vi "TEB.vi"() -> ()   [LabVIEW 2019]
doc: "This is the Target Event Builder (TEB). It basically sits around and waits for event fragments to come in. Each fragment also has an event number attached to it. The TEB stores all fragments indexded by their associated eventnum.\nThe TEB sends fragments to any module appearing in the TEB config file's list. Each destination module can specify what fragments it wants and when those fragments should be sent. The \"when\" decision is made by the TEB based on the age of a given event, the age being determined by how many later events have come in.\nFor example, a module that saves data to disk might specify that it wants its data to be sent after it's 2 events old. So once data for event #1 comes in, it sits in the TEB buffer. Next, data for event #2 comes in, but the TEB keeps the event #1 data in its buffer. Only after event #3 is started (thereby making the event #1 data 2 events old) would the TEB ship event #1 to the module. This aging scheme was added when it was realized that some data for a given event (such as on-line analysis results) may be dependent on sucessive events, and therefore the data cannot be saved until those later events have also started to come in."
uses:
  TEB Global.vi
panel:
  out "Module Response":refnum<k4>
  out "Begin Post Processing":refnum<k4>
  out "Previous Event":T1
  out "Current Event":T1
  in  "stop":bool
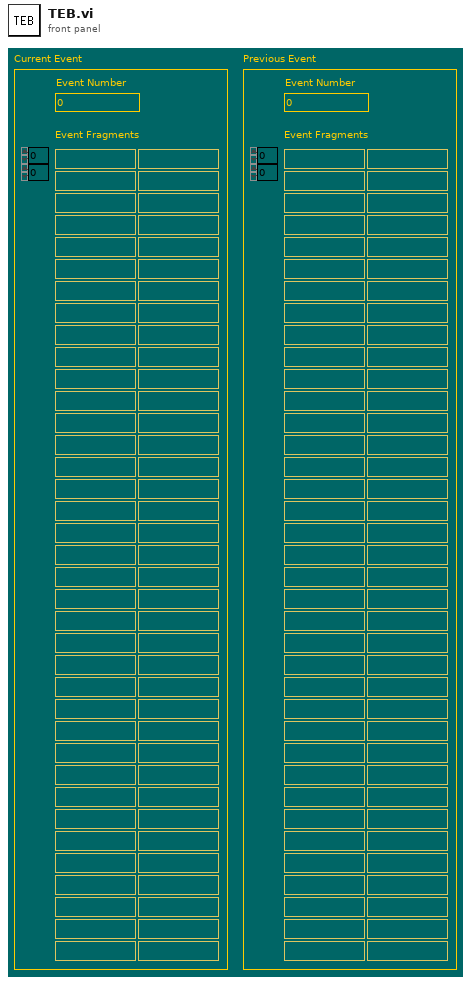
[diagram p1: front panel]
types:
  T1 = cluster{"Event Number":i32, "Event Fragments":string[][]}
  T2 = enum16{"No Message", "Bad Message", "Init", "StartEvent=", "EventFragment=", "InstantFragment=", "StopEvent=", "Processed=", "Address=", "Ping=", "Stop"}
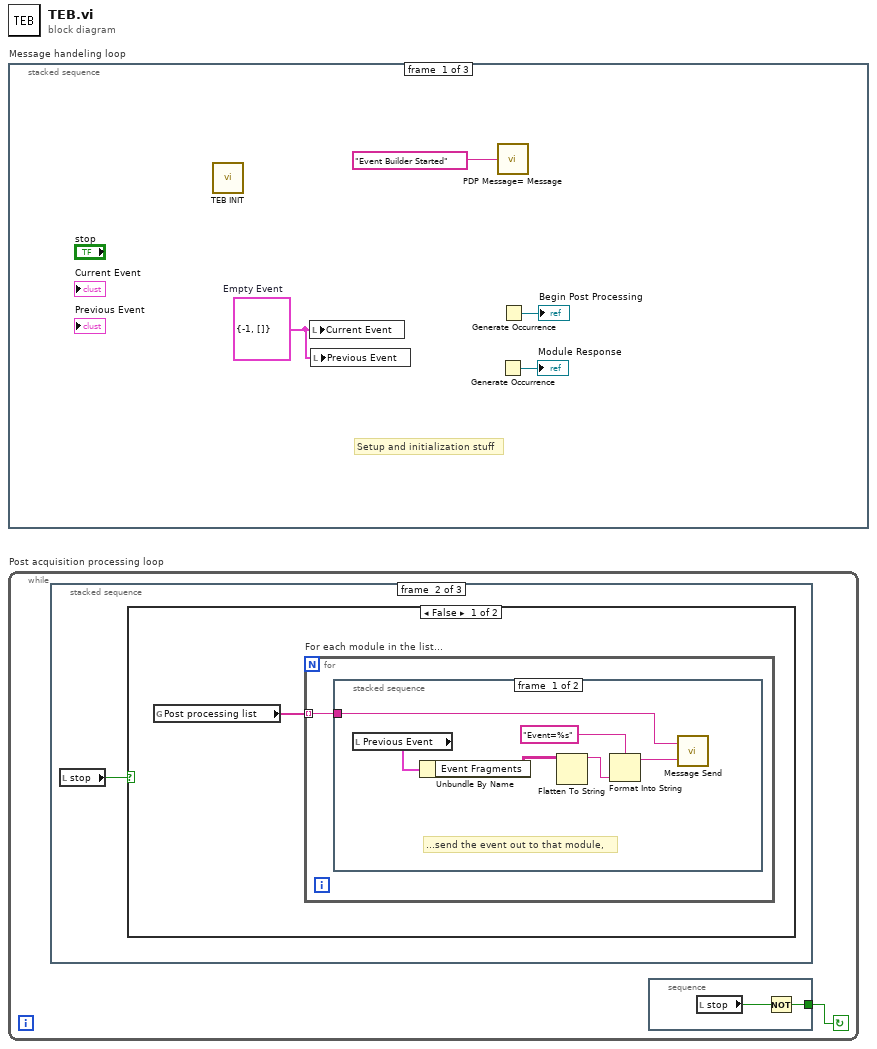
[diagram p0: block diagram]
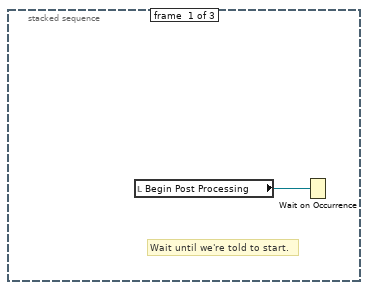
[diagram p2: hidden frame]
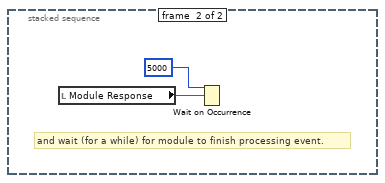
[diagram p3: hidden frame]
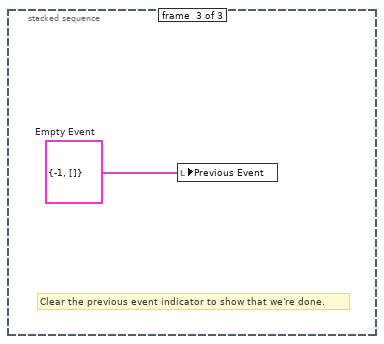
[diagram p5: hidden frame]
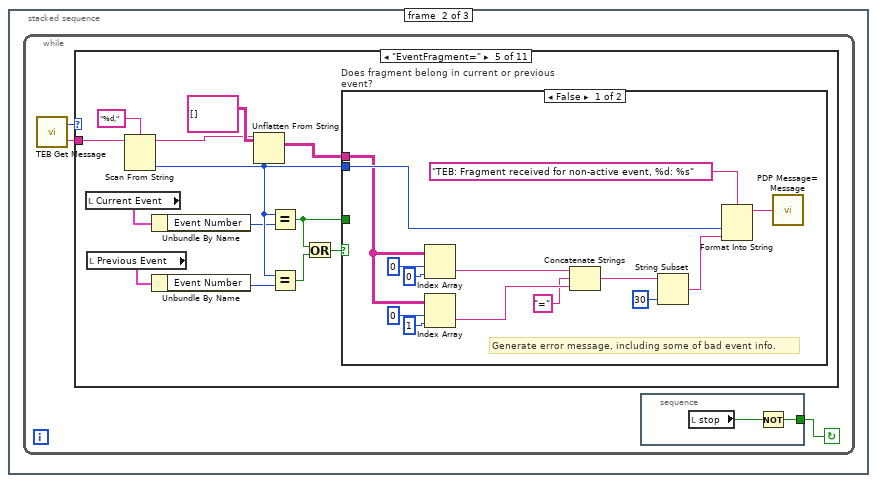
[diagram p6: hidden frame]
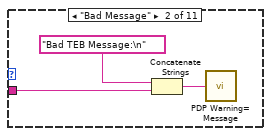
[diagram p8: hidden frame]
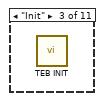
[diagram p9: hidden frame]
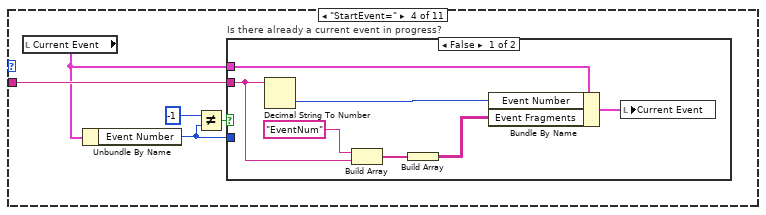
[diagram p10: hidden frame]
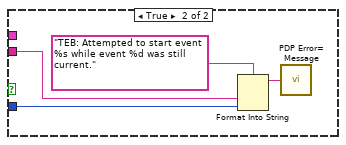
[diagram p11: hidden frame]
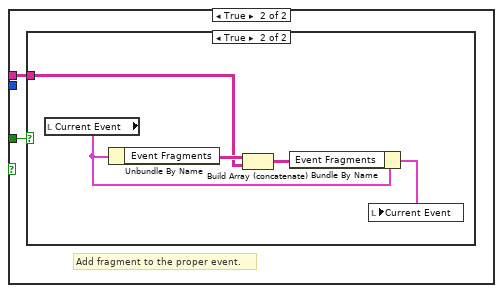
[diagram p12: hidden frame]
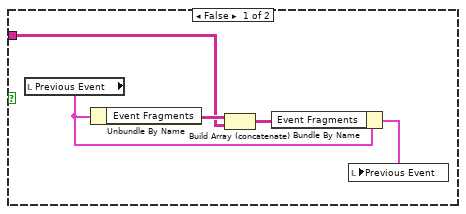
[diagram p13: hidden frame]
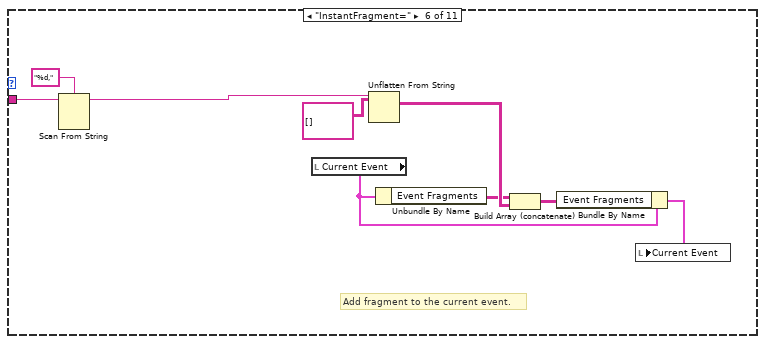
[diagram p14: hidden frame]
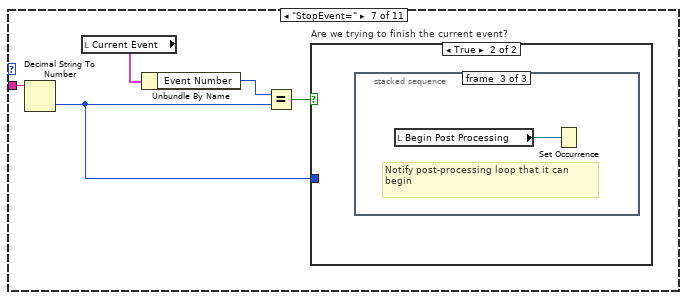
[diagram p15: hidden frame]
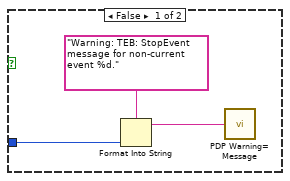
[diagram p16: hidden frame]
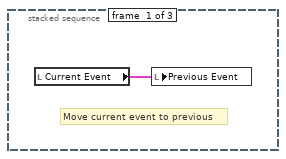
[diagram p17: hidden frame]
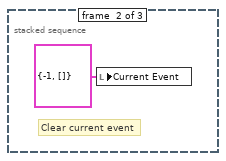
[diagram p18: hidden frame]
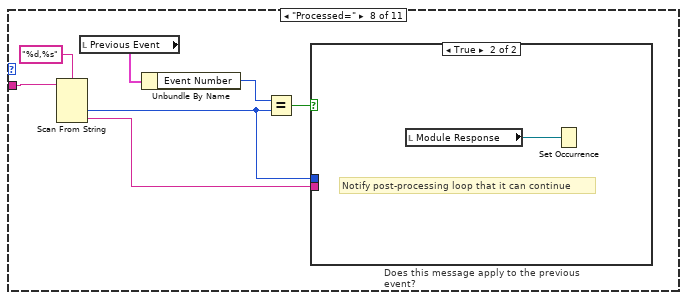
[diagram p19: hidden frame]
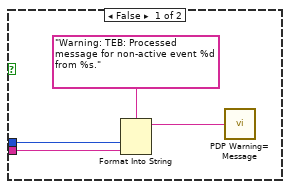
[diagram p20: hidden frame]
diagram:
  n1 = stacked-sequence "Message handeling loop" {
    frame #0 {
      w2 = T1 {"Event Number"=-1, "Event Fragments"=[]}  # Empty Event
      # "Setup and initialization stuff"
      n2 = call "TEB INIT.vi"() -> ()  [unwired: 2 in]
      n3 = local write "Current Event"(w2) -> ()
      n4 = local write "Previous Event"(w2) -> ()
      n5 = call "PDP Message= Message.vi"("Message"="Event Builder Started") -> ()
      n6 = Generate Occurrence() -> (→"Module Response":refnum<k4>)
      n7 = Generate Occurrence() -> (→"Begin Post Processing":refnum<k4>)
    }
    frame #1 {
      n8 = while {
        stop <- w5 continue-if-true
        n9 = call "TEB Get Message.vi"() -> ("Text"=w7:string, "TEB Message Type"=w6:T2)
        n10 = case shown="\"EventFragment=\"" w6 {
          tunnel: w7 -> [_ w12 _ w17 w41 w76 w81 w94 w103 w106 _]
          frame "No Message" {
          }
          frame "Bad Message" {
            n11 = Concatenate Strings("Bad TEB Message:\n", w12) -> (w10:string)
            n12 = call "PDP Warning= Message.vi"("Message"=w10) -> ()
          }
          frame "Init" {
            n13 = call "TEB INIT.vi"() -> ()  [unwired: 2 in]
          }
          frame "StartEvent=" {
            n14 = local read "Current Event"() -> (w16:T1)
            n15 = Unbundle By Name(w16) -> ("Event Number"=w13:i32)
            n16 = Not Equal?(x=-1, y=w13) -> (x != y?=w14:bool)
            n17 = case "Is there already a current event in progress?" shown="False" w14 {
              tunnel: w17 -> [w21 w27]
              tunnel: w16 -> [w22 _]
              tunnel: w13 -> [_ w26]
              frame False {
                n18 = Decimal String To Number(string=w21) -> (number=w24:i32)  [unwired: 2 in, 1 out]
                n19 = Build Array("EventNum", w21) -> (w20:string[])
                n20 = Build Array(w20) -> (w18:string[][])
                n21 = Bundle By Name(cluster=w22, "Event Number"=w24, "Event Fragments"=w18) -> (w23:T1)
                n22 = local write "Current Event"(w23) -> ()
              }
              frame True {
                n23 = Format Into String(format string="TEB: Attempted to start event %s while event %d was still current." ("Format String"), w27, w26) -> (resulting string=w25:string)  [unwired: 2 in, 1 out]
                n24 = call "PDP Error= Message.vi"("Message"=w25) -> ()
              }
            }
          }
          frame "EventFragment=" {
            n25 = local read "Current Event"() -> (w39:T1)
            n26 = local read "Previous Event"() -> (w36:T1)
            n27 = Scan From String(format string="%d,", input string=w41) -> (remaining string=w30:string, output 1=w38:i32)  [unwired: 3 in, 2 out]
            n28 = Unbundle By Name(w39) -> ("Event Number"=w37:i32)
            n29 = Unbundle By Name(w36) -> ("Event Number"=w35:i32)
            n30 = Unflatten From String(type=string[][] [], binary string=w30) -> (value=w29:string[][])  [unwired: 3 in, 2 out]
            n31 = Equal?(x=w38, y=w37) -> (x = y?=w32:bool)
            n32 = Equal?(x=w38, y=w35) -> (x = y?=w34:bool)
            n33 = Or(x=w32, y=w34) -> (x .or. y?=w33:bool)
            n34 = case "Does fragment belong in current or previous event?" shown="False" w33 {
              tunnel: w38 -> [w55 _]
              tunnel: w32 -> [_ w57]
              tunnel: w29 -> [w47 w56]
              frame False {
                # "Generate error message, including some of bad event info."
                n35 = Index Array(array=w47, index (row)=0, index (col)=0 ("disabled index (col)")) -> (element=w44:string)
                n36 = Index Array(array=w47, index (row)=0, index (col)=1 ("disabled index (col)")) -> (element=w43:string)
                n37 = Concatenate Strings(w44, "=" ("string"), w43) -> (w50:string)
                n38 = String Subset(string=w50, length (rest)=30 ("length (rest)")) -> (substring=w52:string)  [unwired: 1 in]
                n39 = Format Into String(format string="TEB: Fragment received for non-active event, %d: %s", w55, w52) -> (resulting string=w53:string)  [unwired: 2 in, 1 out]
                n40 = call "PDP Message= Message.vi"("Message"=w53) -> ()
              }
              frame True {
                # "Add fragment to the proper event."
                n41 = case shown="True" w57 {
                  tunnel: w56 -> [w58 w63]
                  frame False {
                    n42 = local read "Previous Event"() -> (w60:T1)
                    n43 = Unbundle By Name(w60) -> ("Event Fragments"=w61:string[][])
                    n44 = Build Array (concatenate)(w61, w58) -> (w62:string[][])
                    n45 = Bundle By Name(cluster=w60, "Event Fragments"=w62) -> (w59:T1)
                    n46 = local write "Previous Event"(w59) -> ()
                  }
                  frame True {
                    n47 = local read "Current Event"() -> (w65:T1)
                    n48 = Unbundle By Name(w65) -> ("Event Fragments"=w66:string[][])
                    n49 = Build Array (concatenate)(w66, w63) -> (w67:string[][])
                    n50 = Bundle By Name(cluster=w65, "Event Fragments"=w67) -> (w64:T1)
                    n51 = local write "Current Event"(w64) -> ()
                  }
                }
              }
            }
          }
          frame "InstantFragment=" {
            # "Add fragment to the current event."
            n52 = Scan From String(format string="%d,", input string=w76) -> (remaining string=w74:string)  [unwired: 4 in, 2 out]
            n53 = local read "Current Event"() -> (w69:T1)
            n54 = Unflatten From String(type=string[][] [], binary string=w74) -> (value=w73:string[][])  [unwired: 3 in, 2 out]
            n55 = Unbundle By Name(w69) -> ("Event Fragments"=w70:string[][])
            n56 = Build Array (concatenate)(w70, w73) -> (w72:string[][])
            n57 = Bundle By Name(cluster=w69, "Event Fragments"=w72) -> (w68:T1)
            n58 = local write "Current Event"(w68) -> ()
          }
          frame "StopEvent=" {
            n59 = Decimal String To Number(string=w81) -> (number=w79:i32)  [unwired: 2 in, 1 out]
            n60 = local read "Current Event"() -> (w80:T1)
            n61 = Unbundle By Name(w80) -> ("Event Number"=w78:i32)
            n62 = Equal?(x=w78, y=w79) -> (x = y?=w77:bool)
            n63 = case "Are we trying to finish the current event?" shown="True" w77 {
              tunnel: w79 -> [w83 _]
              frame False {
                n64 = Format Into String(format string="Warning: TEB: StopEvent message for non-current event %d." ("Format String"), w83) -> (resulting string=w82:string)  [unwired: 2 in, 1 out]
                n65 = call "PDP Warning= Message.vi"("Message"=w82) -> ()
              }
              frame True {
                n66 = stacked-sequence {
                  frame #0 {
                    # "Move current event to previous"
                    n67 = local read "Current Event"() -> (w85:T1)
                    n68 = local write "Previous Event"(w85) -> ()
                  }
                  frame #1 {
                    # "Clear current event"
                    n69 = local write "Current Event"(T1 {"Event Number"=-1, "Event Fragments"=[]} ("Current Event")) -> ()
                  }
                  frame #2 {
                    # "Notify post-processing loop that it can begin"
                    n70 = local read "Begin Post Processing"() -> (w87:refnum<k4>)
                    n71 = Set Occurrence(w87) -> ()
                  }
                }
              }
            }
          }
          frame "Processed=" {
            n72 = Scan From String(format string="%d,%s", input string=w94) -> (output 1=w90:i32, output 2=w88:string)  [unwired: 4 in, 3 out]
            n73 = local read "Previous Event"() -> (w93:T1)
            n74 = Unbundle By Name(w93) -> ("Event Number"=w92:i32)
            n75 = Equal?(x=w92, y=w90) -> (x = y?=w91:bool)
            n76 = case "Does this message apply to the previous event?" shown="True" w91 {
              tunnel: w90 -> [w97 _]
              tunnel: w88 -> [w95 _]
              frame False {
                n77 = Format Into String(format string="Warning: TEB: Processed message for non-active event %d from %s." ("Format String"), w97, w95) -> (resulting string=w96:string)  [unwired: 2 in, 1 out]
                n78 = call "PDP Warning= Message.vi"("Message"=w96) -> ()
              }
              frame True {
                # "Notify post-processing loop that it can continue"
                n79 = local read "Module Response"() -> (w99:refnum<k4>)
                n80 = Set Occurrence(w99) -> ()
              }
            }
          }
          frame "Address=" {
            n81 = Scan From String(format string="%s,%[.0-9]:%d" ("Format String"), input string=w103) -> (output 1=w101:string, output 2=w102:string, output 3=w100:i32)  [unwired: 5 in, 3 out]
            n82 = call "Message Set Module Address.vi"("Port"=w100, "Address"=w102, "Module"=w101) -> ()
          }
          frame "Ping=" {
            n83 = call "Get UNIX Time.vi"() -> ("UNIX seconds"=w105:i32)
            n84 = Format Into String(format string="PingResponse=TEB,%d", w105) -> (resulting string=w107:string)  [unwired: 2 in, 1 out]
            n85 = call "Message Send.vi"("Message"=w107, "Destination"=w106) -> ()
          }
          frame "Stop" {
            n86 = stacked-sequence {
              frame #0 {
                n87 = local write "stop"(TRUE ("stop")) -> ()
              }
              frame #1 {
                # "Necessary to get other loop to stop, also."
                n88 = local read "Begin Post Processing"() -> (w110:refnum<k4>)
                n89 = Set Occurrence(w110) -> ()
              }
            }
          }
        }
        n90 = stacked-sequence {
          tunnel: [w8] -> w5
          frame #0 {
            n91 = local read "stop"() -> (w9:bool)
            n92 = Not(x=w9) -> (.not. x?=w8:bool)
          }
        }
      }
    }
    frame #2 {
      # "Shutdown stuff"
      n93 = local write "stop"(FALSE ("stop")) -> ()
      n94 = call "PDP Message= Message.vi"("Message"="TEB Module Stopped") -> ()
    }
  }
  n95 = while "Post acquisition processing loop" {
    stop <- w113 continue-if-true
    n96 = stacked-sequence {
      frame #0 {
        # "Wait until we're told to start."
        n97 = local read "Begin Post Processing"() -> (w114:refnum<k4>)
        n98 = Wait on Occurrence(2:w114) -> ()  [unwired: 2 in, 1 out]
      }
      frame #1 {
        n99 = local read "stop"() -> (w115:bool)
        n100 = case shown="False" w115 {
          frame False {
            n101 = global read "TEB Global.vi" "Post processing list"() -> (w116:string[])
            n102 = for "For each module in the list..." {
              tunnel: w116 -> [w117] mode=indexing
              n103 = stacked-sequence {
                tunnel: w117 -> [w120 _]
                frame #0 {
                  # "...send the event out to that module,"
                  n104 = local read "Previous Event"() -> (w123:T1)
                  n105 = Unbundle By Name(w123) -> ("Event Fragments"=w119:string[][])
                  n106 = Flatten To String(anything=w119) -> (data string=w118:string)  [unwired: 3 in, 2 out]
                  n107 = Format Into String(format string="Event=%s" ("Format String"), w118) -> (resulting string=w121:string)  [unwired: 2 in, 1 out]
                  n108 = call "Message Send.vi"("Message"=w121, "Destination"=w120) -> ()
                }
                frame #1 {
                  # "and wait (for a while) for module to finish processing event."
                  n109 = local read "Module Response"() -> (w125:refnum<k4>)
                  n110 = Wait on Occurrence(2:w125, 3:5000 ("ms timeout (-1)")) -> ()  [unwired: 1 in, 1 out]
                }
              }
            }
          }
          frame True {
            # "Do nothing - we've been told to stop."
          }
        }
      }
      frame #2 {
        w126 = T1 {"Event Number"=-1, "Event Fragments"=[]}  # Empty Event
        # "Clear the previous event indicator to show that we're done."
        n111 = local write "Previous Event"(w126) -> ()
      }
    }
    n112 = stacked-sequence {
      tunnel: [w127] -> w113
      frame #0 {
        n113 = local read "stop"() -> (w128:bool)
        n114 = Not(x=w128) -> (.not. x?=w127:bool)
      }
    }
  }
